vi "RSZVB Get Permanent Signal Generator State.vi"(7 "Generator Number (1)":i32=1, 8 "error in (no error)":errorcluster {"code" format="%.0x"}, 9 "Port (1)":i32=1, 10 "Channel (1)":i32=1, 11 "VISA session":refnum<visa-resource-name>) -> (0 "error out":errorcluster {"code" format="%.0x"}, 2 "State":bool, 3 "dup VISA session":refnum<visa-resource-name>)   [LabVIEW 2011]
doc: "This VI queries whether the external generator power is permanently on. \n\nNote(s):\n\n(1) This VI is available only on R&S ZVA instrument.\n\nRemote-control command(s):\nSOURce<Ch>:POWer<Pt>:GENerator<Gen>:PERManent[:STATe]?"
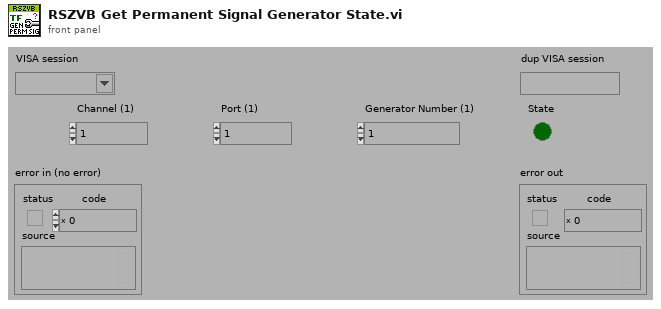
[diagram p1: front panel]
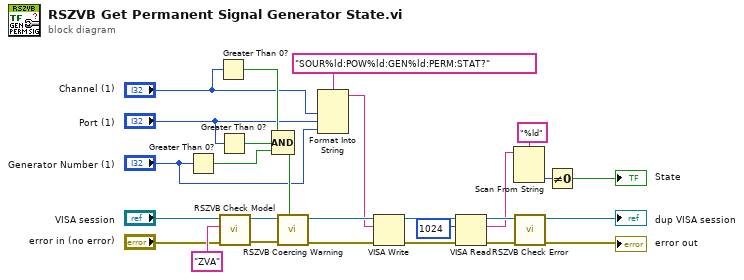
[diagram p0: block diagram]
diagram:
  n1 = Greater Than 0?(x="Generator Number (1)") -> (x > 0?=w7:bool)
  n2 = Greater Than 0?(x="Channel (1)") -> (x > 0?=w22:bool)
  n3 = Greater Than 0?(x="Port (1)") -> (x > 0?=w13:bool)
  n4 = call "RSZVB Check Model.vi"("error in (no error)"="error in (no error)", "Model"="ZVA" ("Options"), "VISA session"="VISA session") -> ("error out"=w1:errorcluster, "dup VISA session"=w2:refnum<visa-resource-name>)  [unwired: 7 in]
  n5 = Compound Arithmetic op=AND(w22, w13, w7) -> (w24:bool)
  n6 = call "RSZVB Coercing Warning.vi"("In Range?"=w24, "error in (no error)"=w1, "VISA session"=w2) -> ("error out"=w25:errorcluster, "dup VISA session"=w26:refnum<visa-resource-name>)  [unwired: 7 in]
  n7 = Format Into String(format string="SOUR%ld:POW%ld:GEN%ld:PERM:STAT?", "Channel (1)", "Port (1)", "Generator Number (1)") -> (resulting string=w23:string)  [unwired: 2 in, 1 out]
  n8 = VISA Write(VISA resource name=w26, write buffer=w23, error in (no error)=w25) -> (VISA resource name out=w15:refnum<visa-resource-name>, error out=w16:errorcluster)  [unwired: 1 out]
  n9 = VISA Read(VISA resource name=w15, byte count=u32 1024 ("byte count (0)"), error in (no error)=w16) -> (VISA resource name out=w20:refnum<visa-resource-name>, read buffer=w18:string, error out=w19:errorcluster)  [unwired: 1 out]
  n10 = Scan From String(format string="%ld", input string=w18) -> (output 1=w17:i32)  [unwired: 3 in, 3 out]
  n11 = call "RSZVB Check Error.vi"("error in (no error)"=w19, "VISA session"=w20) -> ("error out"=→"error out":errorcluster, "dup VISA session"=→"dup VISA session":refnum<visa-resource-name>)  [unwired: 8 in]
  n12 = Not Equal To 0?(x=w17) -> (x != 0?=→"State":bool)
